vi "MGCC_FntStaMach_system_time.vi"   [LabVIEW 2016]
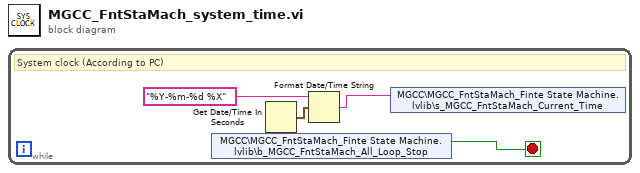
[diagram p0: block diagram]
diagram:
  n1 = while {
    stop <- w2 stop-if-true
    # "System clock (According to PC)"
    n2 = shared-variable "MGCC\\MGCC_FntStaMach_Finte State Machine.lvlib\\b_MGCC_FntStaMach_All_Loop_Stop"() -> (w2:bool)  [unwired: 1 in, 1 out]
    n3 = Get Date/Time In Seconds() -> (seconds since 1Jan1904=w4:timestamp)
    n4 = Format Date/Time String(time format string (%c)="%Y-%m-%d %X", seconds (now)=w4) -> (date/time string=w1:string)  [unwired: 1 in]
    n5 = shared-variable "MGCC\\MGCC_FntStaMach_Finte State Machine.lvlib\\s_MGCC_FntStaMach_Current_Time"(w1) -> ()  [unwired: 1 in, 1 out]
  }
